vi "Unflatten Value.vi"(8 "error in (no error)":errorcluster, 10 "Value":string, 11 "Boolean in":refnum<class "Double 1D.lvclass">) -> (0 "error out":errorcluster, 3 "Boolean out":refnum<class "Double 1D.lvclass">)   [LabVIEW 2019, in "Double 1D.lvclass"]
uses:
  <vilib>/gpm_packages/@cs/data-type-serializer/source/Double 1D/Double 1D.lvclass
  <vilib>/gpm_packages/@cs/data-type-serializer/source/Double 1D/Double 1D.lvclass/Double 1D.ctl
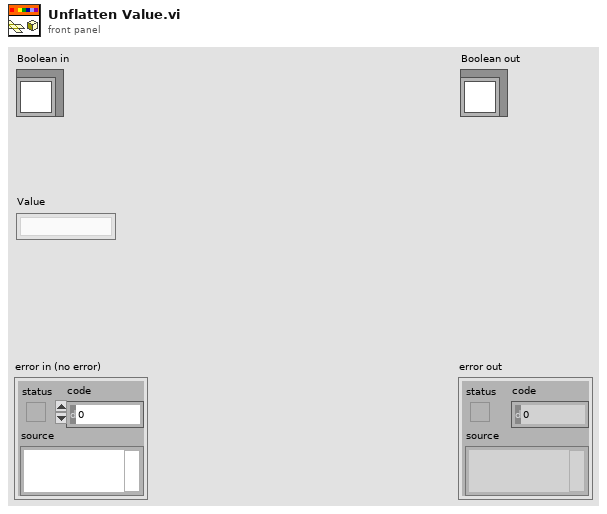
[diagram p1: front panel]
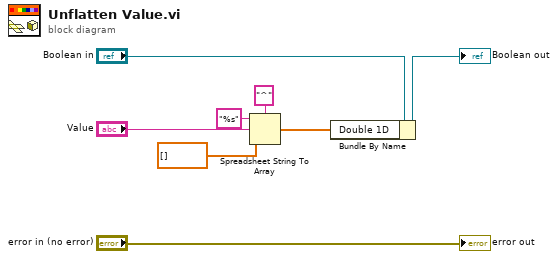
[diagram p0: block diagram]
diagram:
  n1 = Spreadsheet String To Array(delimiter (Tab)="^", format string="%s", spreadsheet string="Value", array type (2D Dbl)=dbl[] [] ("Double 1D")) -> (array=w1:dbl[])
  n2 = Bundle By Name(cluster="Boolean in", "Double 1D"=w1) -> (→"Boolean out":refnum<class "Double 1D.lvclass">)
  "error out" <- "error in (no error)"
